vi "Module Type.vi"(11 "PluginGUI in":refnum<class "PluginGUI.lvclass">) -> (2 "Module Type":string)   [LabVIEW 2020, in "VolatusGUI.lvlib" / "PluginGUI.lvclass"]
uses:
  PluginGUI.lvclass
  PluginGUI.lvclass/PluginGUI.ctl
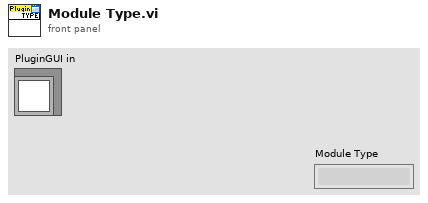
[diagram p1: front panel]
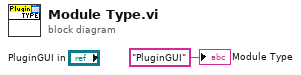
[diagram p0: block diagram]
diagram:
  "Module Type" <- "PluginGUI" ("Module Type")
